vi "Auto Drive Emulation.vi"() -> ()   [LabVIEW 2012]
panel:
  in  "Autonomous Normal":bool
  in  "Autonomous Holonomic":bool
  in  "Autonomous Shooting":bool
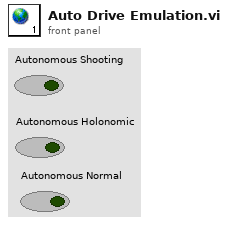
[diagram p1: front panel]
diagram:
